vi "Create Notifiers.vi"(8 "error in":errorcluster) -> (0 "error out":errorcluster, 3 "Notifiers":T1)   [LabVIEW 2020]
uses:
  Notifiers.ctl
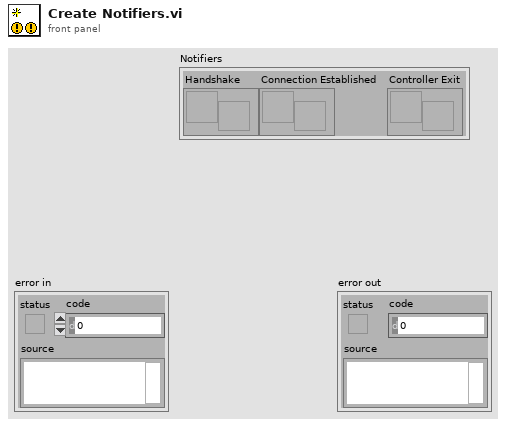
[diagram p1: front panel]
types:
  T1 = typedef "Notifiers.ctl" = cluster{"Handshake":refnum<notifier>, "Connection Established":refnum<notifier>, "Controller Exit":refnum<notifier>}
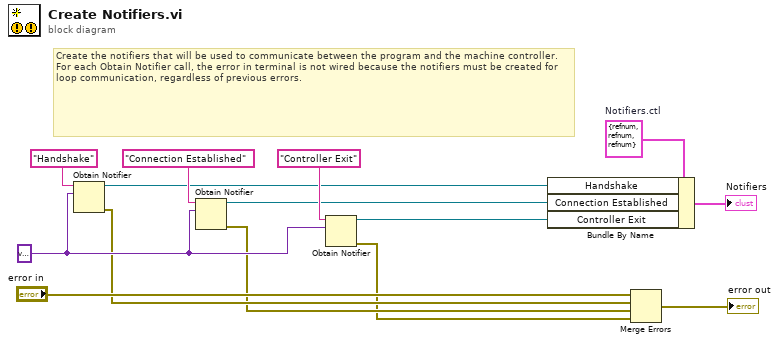
[diagram p0: block diagram]
diagram:
  w10 = T1 {"Handshake"=refnum, "Connection Established"=refnum, "Controller Exit"=refnum}  # Notifiers.ctl
  w11 = variant ("element data type")
  # "Create the notifiers that will be used to communicate between the program and the machine controller. For each Obtain Notifier call, the error in terminal is not wired because the notifiers must be created for loop communication, regardless of previous errors."
  n1 = Obtain Notifier(name (unnamed)="Handshake", notification data type=w11) -> (notifier out=w7:refnum<notifier>, error out=w3:errorcluster)  [unwired: 2 in, 1 out]
  n2 = Obtain Notifier(name (unnamed)="Connection Established", notification data type=w11) -> (notifier out=w8:refnum<notifier>, error out=w2:errorcluster)  [unwired: 2 in, 1 out]
  n3 = Obtain Notifier(name (unnamed)="Controller Exit", notification data type=w11) -> (notifier out=w9:refnum<notifier>, error out=w1:errorcluster)  [unwired: 2 in, 1 out]
  n4 = Bundle By Name(cluster=w10, "Handshake"=w7, "Connection Established"=w8, "Controller Exit"=w9) -> (→"Notifiers":T1)
  n5 = Merge Errors("error in", w3, w2, w1) -> (→"error out":errorcluster)
